vi "add button action.vi"(6 "user event":T1, 8 "error in":errorcluster, 9 "channel list":refnum<vi>, 10 "Engine Configuration":refnum<class "engine configuration.lvclass">, 11 "EIP Tags Configuration in":refnum<class "EIP Tags Configuration.lvclass">) -> (0 "error out":errorcluster, 2 "Engine Configuration out":refnum<class "engine configuration.lvclass">, 3 "module configuration out":refnum<class "EIP Tags Configuration.lvclass">)   [LabVIEW 2013, in "EIP Tags editor node.lvclass"]
uses:
  EIP Tags editor node.lvclass
  <vilib>/NI/TBM Modules/EIP Tags/configuration/EIP Tags Configuration.lvclass
  <vilib>/CEF_TreeControl/Node/UserEventRef.ctl
  <vilib>/CEF_TreeControl/Controls/EventCluster.ctl
  <vilib>/NI/Module Execution Interface/Engine Configuration/engine configuration.lvclass
  <vilib>/NI/Tag Bus Module Framework/root configuration/TBM configuration.lvclass/TBM configuration.ctl
  <vilib>/NI/TBM Modules/EIP Tags/configuration/EIP Tags Configuration.lvclass/EIP Tags Configuration.ctl
  <vilib>/NI/Tag Bus/tag/tag descriptor.lvclass/tag descriptor.ctl
  <vilib>/NI/Tag Bus/tag/write tag name.vi
  <vilib>/NI/TBM Modules/EIP Tags/configuration/Read EIP tags.vi
  <vilib>/NI/Tag Bus Module Framework/root configuration/create GUID.vi
  <vilib>/CEF_TreeControl/NISE_CEF_TreeControl.lvlib
  <vilib>/NI/TBM Modules/EIP Tags/channel/EIP Tags Channel.lvclass
  <vilib>/NI/Tag Bus Module Framework/root configuration/TBM configuration.lvclass
  <vilib>/CEF_TreeControl/Node/NISE_CEF_Node.lvclass
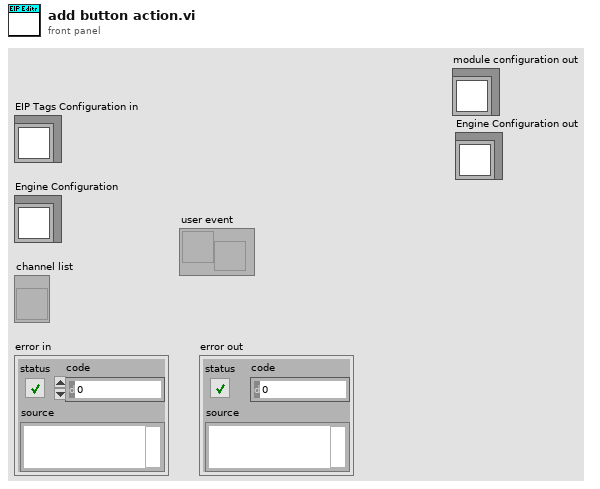
[diagram p1: front panel]
types:
  T1 = typedef "NISE_CEF_Node.lvclass/UserEventRef.ctl" = refnum<user-event>
  T2 = typedef "EIP Tags Configuration.lvclass/eip tag definition.ctl" = cluster{"eip tag types":T3, "unique tag name":string, "Number of Elements":u32}
  T3 = typedef "EIP Tags Configuration.lvclass/eip tag types.ctl" = enum16{"SINT", "INT", "DINT", "REAL", "BOOL", "STRING"}
  T4 = typedef "NISE_CEF_TreeControl.lvlib/EventCluster.ctl" = cluster{"command":string, "data":string}
  T5 = typedef "EIP Tags editor node.lvclass/table line.ctl" = cluster{"eip channel":refnum<class "EIP Tags Channel.lvclass">, "tag name":string}
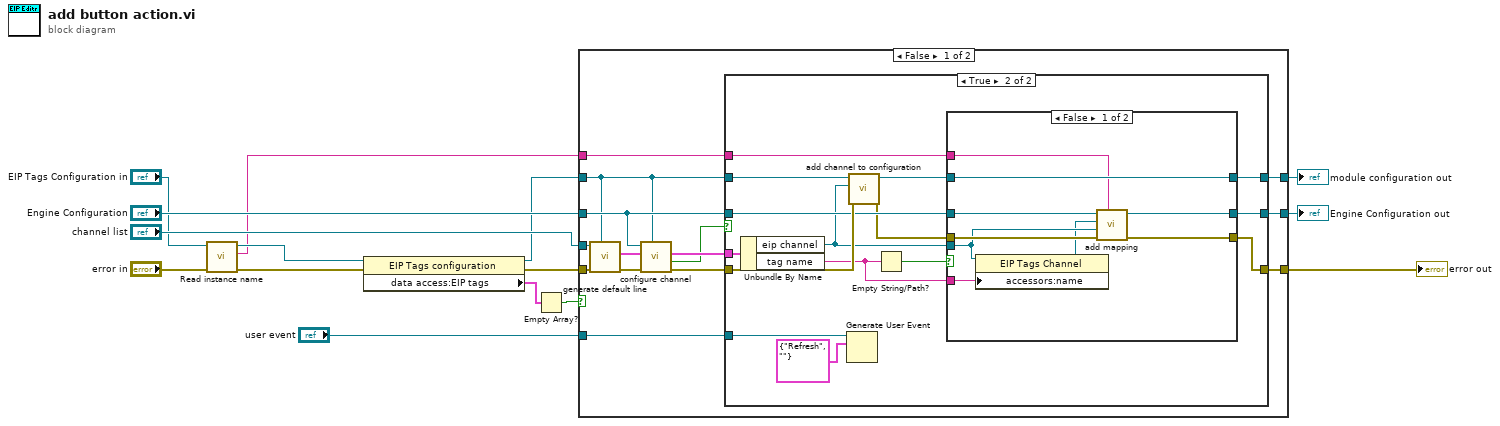
[diagram p0: block diagram]
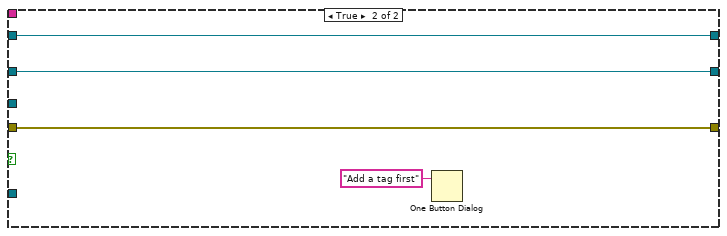
[diagram p4: hidden frame]
diagram:
  n1 = call <vilib>:"Read instance name.vi"("error in"="error in", "configuration in"="EIP Tags Configuration in") -> ("error out"=w7:errorcluster, "instance id"=w4:string, "configuration out"=w5:refnum<class "EIP Tags Configuration.lvclass">)  [unwired: 7 in]
  n2 = property class="EIP Tags configuration"(reference=w5, error in=w7) -> (reference out=w3:refnum<class "EIP Tags Configuration.lvclass">, error out=w13:errorcluster, "data access:EIP tags"=w14:T2[])
  n3 = Empty Array?(array=w14) -> (empty?=w12:bool)
  n4 = case shown="False" w12 {
    tunnel: [w29 w62] -> w8
    tunnel: w13 -> [w28 w62]
    tunnel: "channel list" -> [w27 _]
    tunnel: w3 -> [w17 w60]
    tunnel: "Engine Configuration" -> [w18 w61]
    tunnel: [w22 w61] -> w2
    tunnel: [w21 w60] -> w1
    tunnel: "user event" -> [w19 _]
    tunnel: w4 -> [w16 _]
    frame False {
      n5 = call "generate default line.vi"("EthernetIP configuration"=w17, "error in"=w28, "operations table"=w27) -> ("error out"=w25:errorcluster, "line"=w26:T5)  [unwired: 7 in]
      n6 = call "configure channel.vi"("EthernetIP configuration"=w17, "error in"=w25, "line item in"=w26, "engine configuration in"=w18) -> ("error out"=w23:errorcluster, "success"=w20:bool, "line item out"=w24:T5)  [unwired: 4 in, 1 out]
      n7 = case shown="True" w20 {
        tunnel: [w32 w36] -> w29
        tunnel: w23 -> [w32 w45]
        tunnel: w18 -> [w31 w43]
        tunnel: w24 -> [_ w46]
        tunnel: w17 -> [w30 w47]
        tunnel: [w31 w42] -> w22
        tunnel: [w30 w37] -> w21
        tunnel: w19 -> [_ w35]
        tunnel: w16 -> [_ w33]
        frame False {
        }
        frame True {
          n8 = Unbundle By Name(w46) -> ("eip channel"=w40:refnum<class "EIP Tags Channel.lvclass">, "tag name"=w39:string)
          n9 = Generate User Event(user event=w35, event data cluster=T4 {"command"="Refresh", "data"=""} ("event data")) -> ()  [unwired: 2 in, 2 out]
          n10 = call <vilib>:"add channel to configuration.vi"("error in"=w45, "TBM channel in"=w40, "EthernetIP configuration in"=w47) -> ("error out"=w41:errorcluster, "EthernetIP configuration out"=w38:refnum<class "EIP Tags Configuration.lvclass">)  [unwired: 7 in]
          n11 = Empty String/Path?(string/path=w39) -> (empty?=w44:bool)
          n12 = case shown="False" w44 {
            tunnel: w43 -> [w56 w59]
            tunnel: [w55 w59] -> w42
            tunnel: w41 -> [w54 w58]
            tunnel: w40 -> [w53 _]
            tunnel: w39 -> [w52 _]
            tunnel: [w50 w58] -> w36
            tunnel: w38 -> [w49 w57]
            tunnel: [w49 w57] -> w37
            tunnel: w33 -> [w48 _]
            frame False {
              n13 = property class="EIP Tags Channel"(reference=w53, "accessors:name"=w52) -> (reference out=w51:refnum<class "EIP Tags Channel.lvclass">)  [unwired: 1 in, 1 out]
              n14 = call <vilib>:"add mapping.vi"("owner ID"=w48, "error in"=w54, "channel"=w53, "tag descriptor"=w51, "engine configuration"=w56) -> ("error out"=w50:errorcluster, "engine configuration out"=w55:refnum<class "engine configuration.lvclass">)  [unwired: 5 in]
            }
            frame True {
            }
          }
        }
      }
    }
    frame True {
      n15 = One Button Dialog(message="Add a tag first") -> ()  [unwired: 1 in, 1 out]
    }
  }
  "error out" <- w8
  "Engine Configuration out" <- w2
  "module configuration out" <- w1
